vi "Helper SubVI - Simulate Multiplexed Signals.vi"(8 "error in (no error)":errorcluster, 9 "#channels":i32=4, 10 "sampling info":cluster{"Fs":dbl, "#s":dbl}={"Fs"=1000.0, "#s"=1000.0} {"Fs" format="%.2p"}, 11 "frequency":dbl=10.0 format="%#.6g") -> (0 "error out":errorcluster, 3 "signal array out":waveform(dbl)[](array[waveform]))   [LabVIEW 2020]
doc: "Simulates data acquired through a multiplexer. Each channel is offset by a multiple of dt."
uses:
  <vilib>/measure/NI_MABase.lvlib
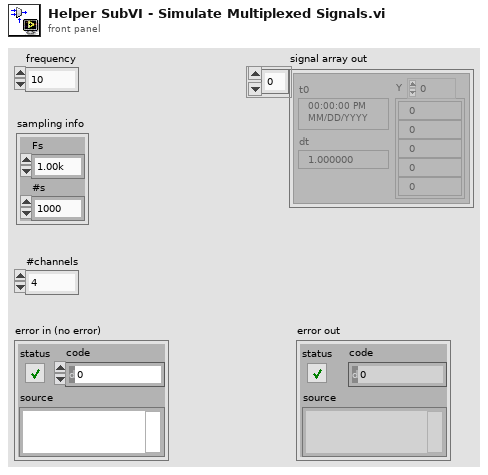
[diagram p1: front panel]
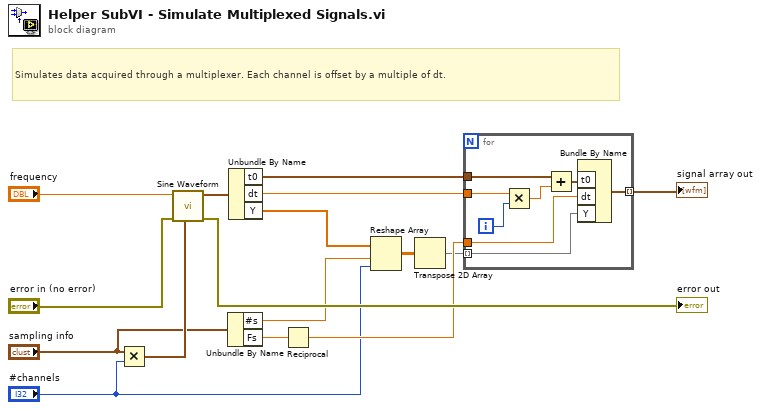
[diagram p0: block diagram]
diagram:
  # "Simulates data acquired through a multiplexer. Each channel is offset by a multiple of dt."
  n1 = Multiply(x="sampling info", y="#channels") -> (x*y=w5:cluster{"Fs":dbl, "#s":dbl})
  n2 = call <vilib>:"Sine Waveform.vi"("sampling info"=w5, "error in (no error)"="error in (no error)", "frequency"="frequency") -> ("error out"=→"error out":errorcluster, "signal out"=w13:waveform(dbl))  [unwired: 4 in, 3 out]
  n3 = Unbundle By Name("sampling info") -> ("#s"=w2:dbl, "Fs"=w10:dbl)
  n4 = Unbundle By Name(w13) -> ("t0"=w11:timestamp, "dt"=w12:dbl, "Y"=w8:dbl[])
  n5 = Reciprocal(x=w10) -> (1/x=w9:dbl)
  n6 = Reshape Array(w8, w2, "#channels") -> (w7:dbl[][])
  n7 = Transpose 2D Array(2D array=w7) -> (transposed array=w1:dbl[][])
  n8 = for {
    tunnel: w12 -> [w21]
    tunnel: w11 -> [w24]
    tunnel: w9 -> [w20]
    tunnel: w1 -> [w19] mode=indexing
    tunnel: [w18] -> w6 mode=indexing
    i -> [w22]
    n9 = Multiply(x=w21, y=w22) -> (x*y=w23:dbl)
    n10 = Add(x=w24, y=w23) -> (x+y=w17:timestamp)
    n11 = Bundle By Name("t0"=w17, "dt"=w20, "Y"=w19) -> (w18:waveform(dbl))  [unwired: 1 out]
  }
  "signal array out" <- w6
